vi "3D-DownLoadPath.vi"(8 "名称或相对路径":string, 11 "路径":path) -> (3 "VersionParams":string[][](array[string]) caption="所有行")   [LabVIEW 2015]
uses:
  <vilib>/Utility/file.llb/Read From Spreadsheet File (string).vi
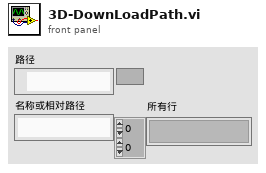
[diagram p1: front panel]
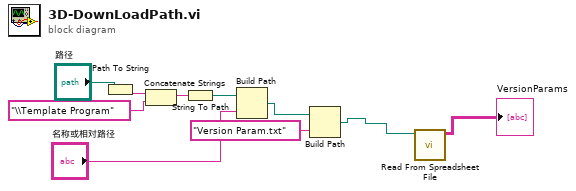
[diagram p0: block diagram]
diagram:
  n1 = Path To String(path="路径") -> (string=w10:string)
  n2 = Concatenate Strings(w10, "\\Template Program" ("字符串")) -> (w9:string)
  n3 = String To Path(string=w9) -> (path=w7:path)
  n4 = Build Path(base path=w7, name or relative path="名称或相对路径") -> (appended path=w4:path)
  n5 = Build Path(base path=w4, name or relative path="Version Param.txt" ("名称或相对路径")) -> (appended path=w2:path)
  n6 = call-poly <vilib>:"Read From Spreadsheet File.vi"("file path (dialog if empty)"=w2) -> ("all rows"=→"VersionParams":string[][])  [unwired: 6 in, 4 out]
